vi "New DAC8552.vi"(8 "error in (no error)":errorcluster, 9 "VRef (5V)":dbl=5.0, 10 "SPI CS Line":u8=15, 11 "SPI in":refnum<class "LINX SPI.lvclass">) -> (0 "error out":errorcluster, 3 "LINX-DAC8552 out":refnum<class "LINX-DAC8552.lvclass">)   [LabVIEW 2020, in "LINX-DAC8552.lvclass"]
doc: "Creates a new instance of a DAC8552 device from the SPI configuration."
uses:
  LINX-DAC8552.lvclass
  LINX SPI/LINX SPI.lvclass
  <vilib>/MakerHub/LINX/Public/Peripherals/SPI/SPI CS Config.ctl
  <vilib>/MakerHub/LINX/Private/Type Defs/Peripherals/SPI/SPI CS Logic Level.ctl
  LINX SPI/LINX SPI.lvclass/LINX SPI.ctl
  LINX-DAC8552.lvclass/LINX-DAC8552.ctl
  LINX SPI/Write CS Configuration.vi
  Write SPI.vi
  Write VRef.vi
  <vilib>/MakerHub/LINX/LMH-LINX.lvlib
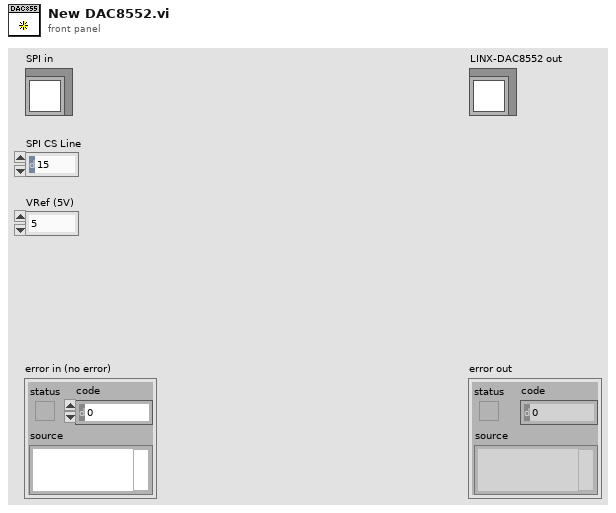
[diagram p1: front panel]
types:
  T1 = typedef "LMH-LINX.lvlib/SPI CS Config.ctl" = cluster{"CS Channel":u8, "CS Logic Level":T2}
  T2 = typedef "LMH-LINX.lvlib/SPI CS Logic Level.ctl" = enum8{"Active Low", "Active High"}
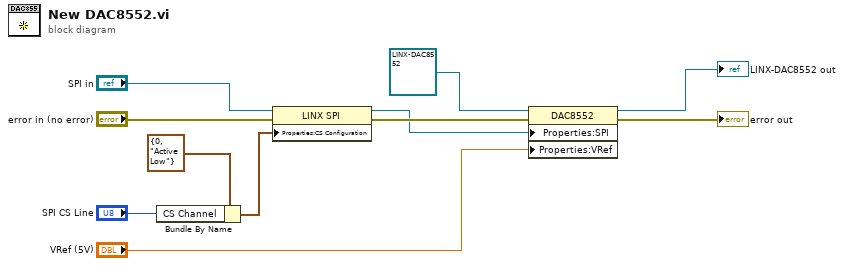
[diagram p0: block diagram]
diagram:
  n1 = Bundle By Name(cluster=T1 {"CS Channel"=0, "CS Logic Level"=enum."Active Low"} ("CS Configuration"), "CS Channel"="SPI CS Line") -> (w2:T1)
  n2 = property class="LINX SPI"(reference="SPI in", error in="error in (no error)", "Properties:CS Configuration"=w2) -> (reference out=w1:refnum<class "LINX SPI.lvclass">, error out=w6:errorcluster)
  n3 = property class="DAC8552"(reference=refnum<class "LINX-DAC8552.lvclass"> refnum ("LINX-DAC8552 out"), error in=w6, "Properties:SPI"=w1, "Properties:VRef"="VRef (5V)") -> (reference out=→"LINX-DAC8552 out":refnum<class "LINX-DAC8552.lvclass">, error out=→"error out":errorcluster)
